vi "Log Warning.vi"(4 "User":string, 6 "Level":string, 8 "error in":errorcluster, 10 "Message":string, 11 "Data":refnum<class "Logging Service.lvclass">) -> (0 "error out":errorcluster)   [LabVIEW 2026, in "Logging Service.lvclass"]
uses:
  Logging Service.lvclass
  Logging Service.lvclass/Logging Service.ctl
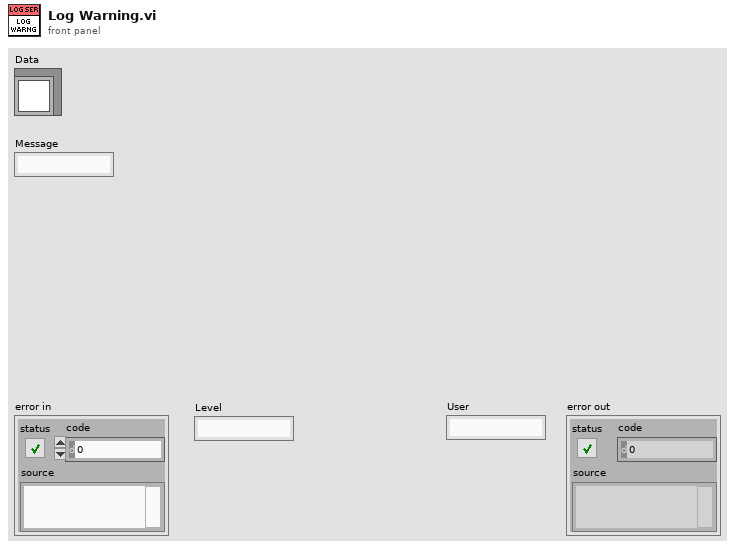
[diagram p1: front panel]
types:
  T1 = enum16{"open", "replace", "create", "open or create", "replace or create", "replace or create with confirmation"}
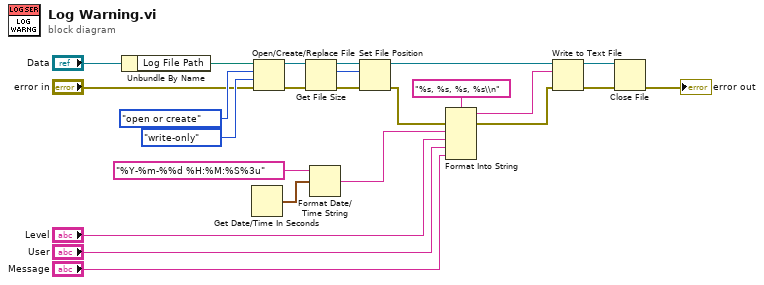
[diagram p0: block diagram]
diagram:
  n1 = Unbundle By Name("Data") -> ("Log File Path"=w21:path)
  n2 = Get Date/Time In Seconds() -> (seconds since 1Jan1904=w24:timestamp)
  n3 = Open/Create/Replace File(file path (use dialog)=w21, error in="error in", operation (0:open)=T1."open or create", access (0:read/write)=enum16{"read/write", "read-only", "write-only"}."write-only") -> (refnum out=w17:refnum<file>, error out=w16:errorcluster)  [unwired: 2 in, 1 out]
  n4 = Get File Size(file=w17, error in=w16) -> (refnum out=w15:refnum<file>, size (in bytes)=w13:i64, 0:w14:errorcluster)
  n5 = Format Date/Time String(time format string (%c)="%Y-%m-%%d %H:%M:%S%3u", seconds (now)=w24) -> (date/time string=w5:string)  [unwired: 1 in]
  n6 = Set File Position(offset (in bytes) (0)=w13, refnum=w15, error in=w14) -> (refnum out=w12:refnum<file>, error out=w8:errorcluster)  [unwired: 1 in]
  n7 = Format Into String(format string="%s, %s, %s, %s\\n", error in=w8, w5, "Level", "User", "Message") -> (resulting string=w1:string, error out=w6:errorcluster)  [unwired: 1 in]
  n8 = Write to Text File(file (use dialog)=w12, text=w1, error in=w6) -> (refnum out=w10:refnum<file>, error out=w11:errorcluster)  [unwired: 1 in, 1 out]
  n9 = Close File(refnum=w10, error in=w11) -> (error out=→"error out":errorcluster)  [unwired: 1 out]
